vi "Create Temp.vi"(10 "Path":path) -> (1 "Temporary":path, 2 "Original":path)   [LabVIEW 2019, in "TDMS.lvlib" / "TDMS.lvclass"]
uses:
  TDMS.lvclass
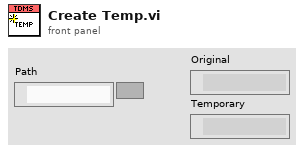
[diagram p1: front panel]
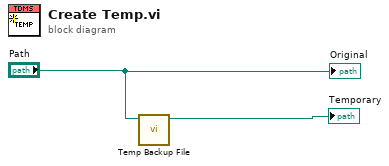
[diagram p0: block diagram]
diagram:
  n1 = call <vilib>:"Temp Backup File.vi"("destination"="Path") -> ("backup"=→"Temporary":path)  [unwired: 8 in, 2 out]
  "Original" <- "Path"
